vi "Nest Msg Send.vi"(7 "Actor":refnum<class "LVCAM.lvclass">, 8 "Alias":string, 9 "Priority Msg?":bool, 10 "Msg":refnum<class "Msg.lvclass">) -> (0 "error out":errorcluster, 2 "Alias found?":bool)   [LabVIEW 2021, in "LVCAM.lvlib" / "Actor.lvclass"]
uses:
  Actor.lvclass
  Msg/Msg.lvclass
  LVCAM/LVCAM.lvclass
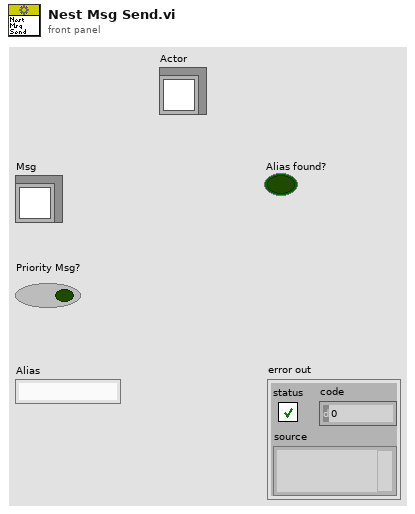
[diagram p1: front panel]
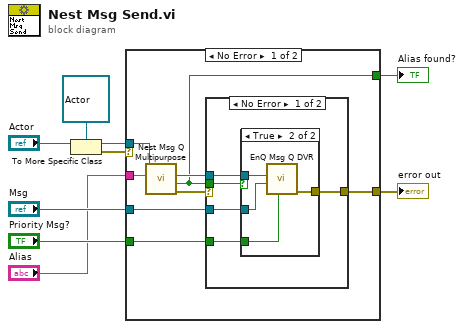
[diagram p0: block diagram]
diagram:
  n1 = To More Specific Class(target class=refnum<class "Actor.lvclass"> refnum ("LVCAM.lvlib:Self Actor.lvclass"), reference="Actor") -> (specific class reference=w5:refnum<class "Actor.lvclass">, error out=w3:errorcluster)  [unwired: 1 in]
  n2 = case shown="No Error" w3 {
    selector: w3 -> [_ w28]
    tunnel: [w17 w28] -> w9
    tunnel: "Msg" -> [w16 _]
    tunnel: "Priority Msg?" -> [w15 _]
    tunnel: w5 -> [w12 _]
    tunnel: "Alias" -> [w13 _]
    tunnel: [w10 _] -> w1
    frame No Error {
      n3 = call "Nest Msg Q Multipurpose.vi"("Alias"=w13, "Actor in"=w12) -> ("error out"=w14:errorcluster, "Alias found?"=w10:bool, "Nest Msg Q"=w11:refnum<data-value>)  [unwired: 5 in, 2 out]
      n4 = case shown="No Error" w14 {
        selector: w14 -> [_ w27]
        tunnel: [w22 w27] -> w17
        tunnel: w16 -> [w21 _]
        tunnel: w15 -> [w20 _]
        tunnel: w10 -> [w19 _]
        tunnel: w11 -> [w18 _]
        frame No Error {
          n5 = case shown="True" w19 {
            tunnel: [_ w23] -> w22
            tunnel: w21 -> [_ w25]
            tunnel: w20 -> [_ w24]
            tunnel: w18 -> [_ w26]
            frame False {
            }
            frame True {
              n6 = call "EnQ Msg Q DVR.vi"("Priority Msg?"=w24, "Msg"=w25, "Msg Q DVR"=w26) -> ("error out"=w23:errorcluster)  [unwired: 8 in]
            }
          }
        }
        frame Error {
          # "#LVCAMError"
        }
      }
    }
    frame Error {
    }
  }
  "error out" <- w9
  "Alias found?" <- w1
